vi "Mutate Configuration to Current.vi"(8 "error in (no error)":errorcluster, 9 "Serialized Version":T2, 10 "Serialized Configuration in":string, 11 "Automated Config Attempt":T1) -> (0 "error out":errorcluster, 3 "Config Out":T1)   [LabVIEW 2020, in "RandomNumberGenerator.lvlib" / "RandomNumberGenerator.lvclass"]
doc: "<b>Mutate Configuration to Current</b>\nThis method is responsible for mutating the configuration data to the latest version."
uses:
  RandomNumberGenerator.lvclass
  RandomNumberGenerator.lvclass/RandomNumberGenerator.ctl
  <vilib>/ADAS Record/Utilities/ADAS Utilities.lvlib
  Configuration.ctl
  <vilib>/ADAS Record/Utilities/TypeDefs/Config Version.ctl
panel:
  # "#via_ignore"
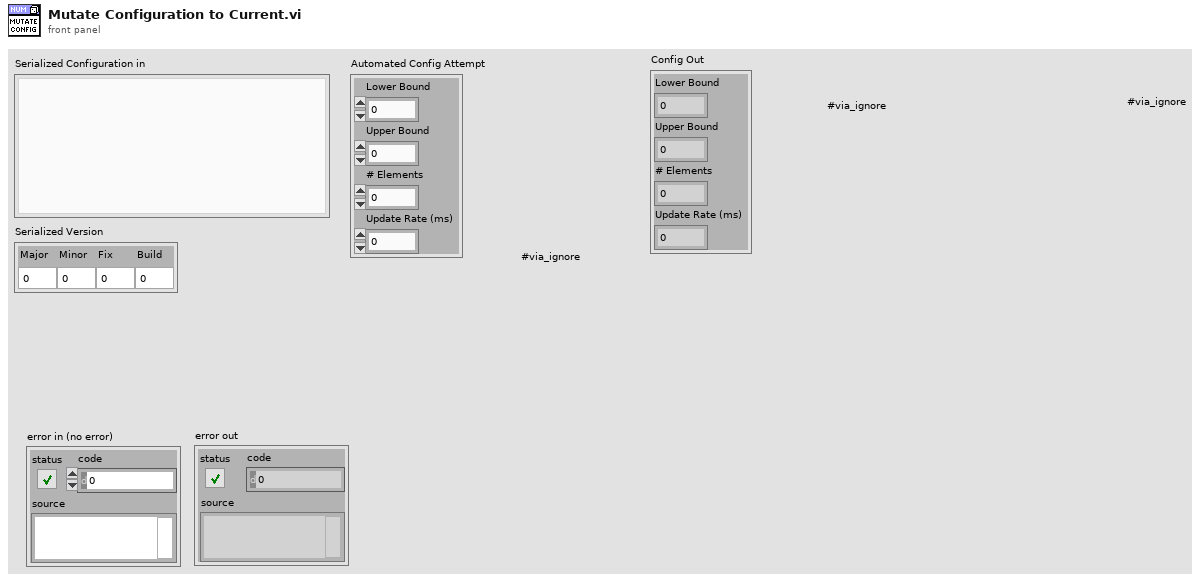
[diagram p1: front panel]
types:
  T1 = typedef "RandomNumberGenerator.lvlib/RandomNumberGenerator.lvclass/Configuration.ctl" = cluster{"Lower Bound":dbl, "Upper Bound":dbl, "# Elements":i32, "Update Rate (ms)":i32}
  T2 = typedef "ADAS Utilities.lvlib/Config Version.ctl" = cluster{"Major":u32, "Minor":u32, "Fix":u32, "Build":u32}
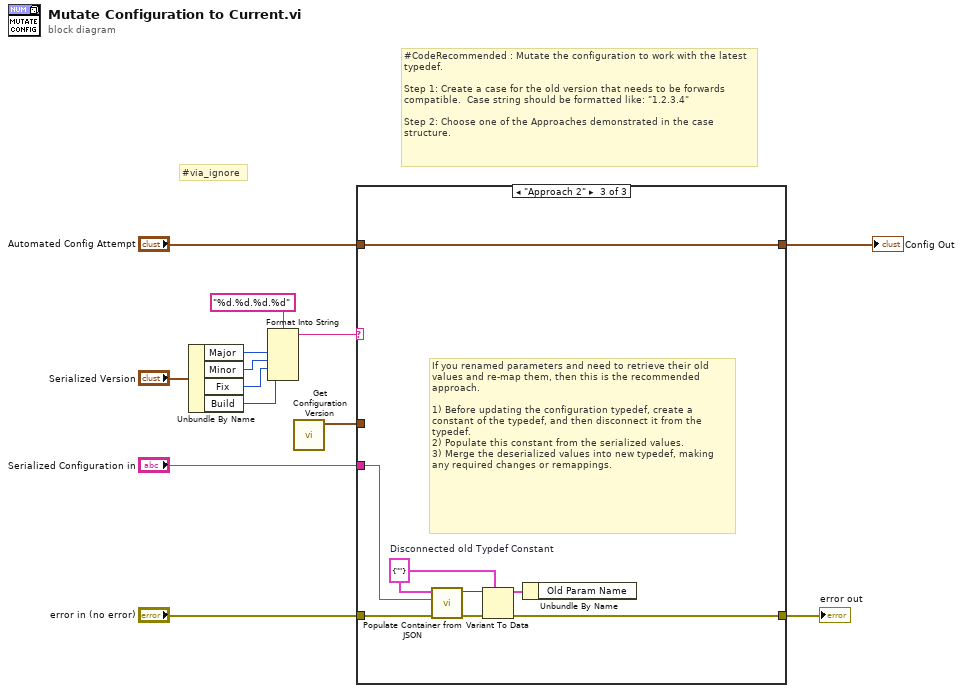
[diagram p0: block diagram]
diagram:
  # "#via_ignore"
  # "#CodeRecommended : Mutate the configuration to work with the latest typedef.\n\nStep 1: Create a case for the old version that needs to be forwards compatible.  Case string should be formatted like: \"1.2.3.4\"\n\nStep 2: Choose one of the Approaches demonstrated in the case structure."
  n1 = Unbundle By Name("Serialized Version") -> ("Major"=w7:u32, "Minor"=w6:u32, "Fix"=w5:u32, "Build"=w4:u32)
  n2 = Format Into String(format string="%d.%d.%d.%d", w7, w6, w5, w4) -> (resulting string=w2:string)  [unwired: 2 in, 1 out]
  n3 = call "Get Configuration Version.vi"() -> ("Version"=w1:T2)  [unwired: 11 in]
  n4 = case shown="\"Approach 2\"" w2 {
    tunnel: "Serialized Configuration in" -> [_ _ w24]
    tunnel: [w15 w16 w19] -> w12
    tunnel: "error in (no error)" -> [w15 w16 w25]
    tunnel: "Automated Config Attempt" -> [w14 w17 w18]
    tunnel: [w14 w17 w18] -> w9
    tunnel: w1 -> [_ _ _]
    frame Default {
    }
    frame "Approach 1" {
      # "If only new parameters have been added, then just use the \"Automated Config Attempt\".  This is the automated attempt at merging old values into the new configuration.  If values have the same names and previously existed, they get set.  If parameters are new in the new config, then their default values will be used."
    }
    frame "Approach 2" {
      w23 = cluster{"Old Param Name":string} {"Old Param Name"=""}  # Disconnected old Typdef Constant
      # "If you renamed parameters and need to retrieve their old values and re-map them, then this is the recommended approach.\n\n1) Before updating the configuration typedef, create a constant of the typedef, and then disconnect it from the typedef.\n2) Populate this constant from the serialized values.\n3) Merge the deserialized values into new typedef, making any required changes or remappings."
      n5 = call <vilib>:"Populate Container from JSON.vi"("error in (no error)"=w25, "JSON string In"=w24, "Container In"=w23) -> ("error out"=w21:errorcluster, "Container Out"=w22:variant)  [unwired: 6 in, 1 out]
      n6 = Variant To Data(error in=w21, type=w23, Variant=w22) -> (data=w20:cluster{"Old Param Name":string}, error out=w19:errorcluster)
      n7 = Unbundle By Name(w20) -> ()  [unwired: 1 out]
    }
  }
  "error out" <- w12
  "Config Out" <- w9
